vi "Limit_Switch.vi"(6 "Echo Mode":i32, 7 "Motor":u16(ring) items=["none", "1", "2", "3", "4", "all"], 8 "error in (no error)":errorcluster, 11 "VISA resource name":refnum<visa-resource-name>) -> (0 "error out":errorcluster={"status"=FALSE, "code"=1073676294, "source"="VISA Read in write_read.vi"}, 1 "Limit Switch min":bool, 2 "Limit Switch max":bool, 3 "VISA ressource out":refnum<visa-resource-name>, 5 "Error?":bool)   [LabVIEW 2018]
uses:
  MCode_LV_86/Set Parameter.ctl
panel:
  out "Value Error":i32
  out "Value Flag":i32
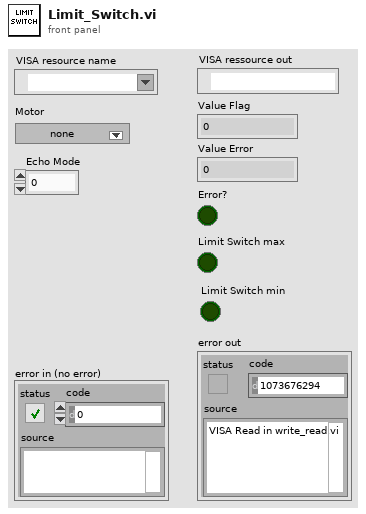
[diagram p1: front panel]
types:
  T1 = typedef "Set Parameter.ctl" = enum16{"Acceleration (A)", "Baud Rate (BD)", "Counter 1 (C1)", "Counter 2 (C2)", "Control C Software Reset (CE)", "Check Sum Enable (CK)", "Clock Mode (CM)", "Clock Mode Ratio (CR)", "Clock Mode Out Step Width (CW)", "Deceleration (D)", "Digital Filtering, Input 1 (D1)", "Digital Filtering, Input 2 (D2)", "Digital Filtering, Input 3 (D3)", "Digital Filtering, Input 4 (D4)", "Digital Filtering, Input 5 (D5)", "Digital Filtering, Input 9 (D9)", "Digital Filtering, Input 10 (D10)", "Digital Filtering, Input 11 (D11)", "Digital Filtering, Input 12 (D12)", "Deadband (DB)", "Decrement Variable (DC)", "Enable/Disable Drive (DE)", "Device Name (DN)", "End Program Execution (E)", "Encoder Function Enable (EE)", "Error Flag (EF)", "Encoder Lines (EL)", "Echo Mode (EM)", "Error Value (ER)", "Escape (ES)", "Execute Program at Address (EX)", "Firmware Version (VR)", "Hold (H)", "Hold Current (HC)", "Hold Current Delay Time (HI)", "Home to Encoder Index (HM)", "Home to Home Switch (HT)", "Increment Variable (IC)", "Initialize Parameters to NVM (IP)", "Input into Variable (IV)", "Jog Enable (JE)", "Limit Stop Mode (LM)", "Move Absolute (MA)", "Move Relative (MR)", "MicroStepping Select (MS)", "Motor Settling Delay Time (MT)", "Moving [Flag] (MV)", "Output 1 (O1)", "Output 2 (O2)", "Output 3 (O3)", "Output 4 (O4)", "Output 9 (O9)", "Output 10 (O10)", "Output 11 (O11)", "Output 12 (O12)", "Output High Byte (9-12) (OH)", "Output Low Byte (1-4) (OL)", "Output Total (1-4 and 9-12) (OT)", "Position (P)", "Position Maintenance (PM)", "Party Mode (PY)", "Register 1 (R1)", "Register 2 (R2)", "Register 3 (R3)", "Register 4 (R4)", "Reset Error(\\03)", "Run Current (RC)", "Stall Factor (SF)", "Slew (SL)", "Stall Mode Set (SM)", "Upgrade Firmware (UG)", "Velocity Initial (VI)", "Velocity Maximum (VM)", "Current1 (I1)", "Current2 (I2)", "Current3 (I3)", "Current4 (I4)", "Current5 (I5)", "Current6 (I6)", "Save (S)"}
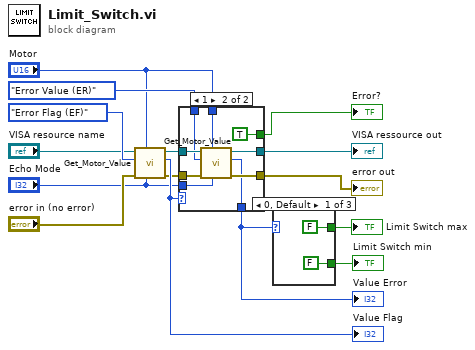
[diagram p0: block diagram]
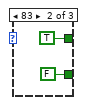
[diagram p2: hidden frame]
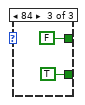
[diagram p3: hidden frame]
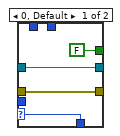
[diagram p4: hidden frame]
diagram:
  n1 = call "Get_Motor_Value.vi"("Echo Mode"="Echo Mode", "Motor"="Motor", "error in (no error)"="error in (no error)", "Command"=Set_Parameter."Error Flag (EF)", "VISA resource name"="VISA resource name") -> ("error out"=w11:errorcluster, "Value"=w12:i32, "VISA ressource out"=w10:refnum<visa-resource-name>)  [unwired: 3 in, 1 out]
  "Value Flag" <- w12
  n2 = case shown="1" w12 {
    selector: w12 -> [w17 _]
    tunnel: w11 -> [w18 w27]
    tunnel: w10 -> [w19 w28]
    tunnel: [w19 w23] -> w5
    tunnel: [w18 w22] -> w6
    tunnel: Set_Parameter."Error Value (ER)" ("Command") -> [_ w26]
    tunnel: "Motor" -> [_ w25]
    tunnel: "Echo Mode" -> [_ w24]
    tunnel: [w17 w21] -> w4
    tunnel: [FALSE TRUE] -> w3
    frame 0, Default {
    }
    frame 1 {
      n3 = call "Get_Motor_Value.vi"("Echo Mode"=w24, "Motor"=w25, "error in (no error)"=w27, "Command"=w26, "VISA resource name"=w28) -> ("error out"=w22:errorcluster, "Value"=w21:i32, "VISA ressource out"=w23:refnum<visa-resource-name>)  [unwired: 3 in, 1 out]
    }
  }
  "error out" <- w6
  "VISA ressource out" <- w5
  "Value Error" <- w4
  "Error?" <- w3
  n4 = case shown="0, Default" w4 {
    tunnel: [FALSE TRUE FALSE] -> w2
    tunnel: [FALSE FALSE TRUE] -> w1
    frame 0, Default {
    }
    frame 83 {
    }
    frame 84 {
    }
  }
  "Limit Switch max" <- w2
  "Limit Switch min" <- w1
